vi "WriteDAQ_2AO.vi"(0 "data":dbl format="%0.2f", 1 "array":cluster{dbl, string, "Output Channels":tag}[](array[cluster]), 2 "Channel":i32=1) -> ()   [LabVIEW 2013]
uses:
  <vilib>/DAQmx/write.llb/DAQmx Write (Analog DBL 1Chan 1Samp).vi
  <vilib>/DAQmx/create/channels.llb/DAQmx Create Channel (AO-Voltage-Basic).vi
  <vilib>/DAQmx/miscellaneous.llb/DAQmx Fill In Error Info.vi
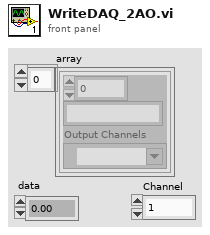
[diagram p1: front panel]
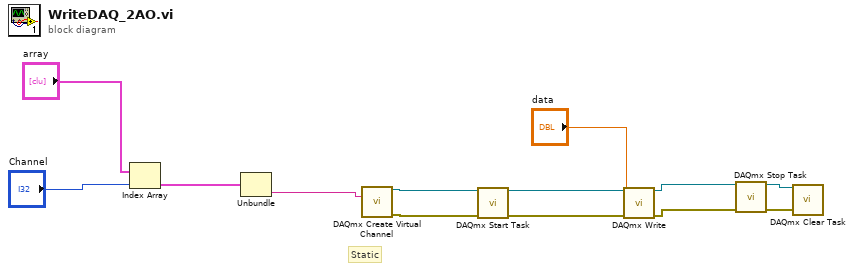
[diagram p0: block diagram]
diagram:
  # "Static"
  n1 = Index Array(array="array", index="Channel") -> (element=w5:cluster{dbl, string, "Output Channels":tag})
  n2 = Unbundle(w5) -> ("Output Channels"=w2:tag)  [unwired: 2 out]
  n3 = call-poly <vilib>:"DAQmx Create Virtual Channel.vi"("physical channels"=w2) -> ("task out"=w6:refnum<k21>, "error out"=w7:errorcluster)  [unwired: 13 in]
  n4 = call <vilib>:"DAQmx Start Task.vi"("task/channels in"=w6, "error in"=w7) -> ("task out"=w8:refnum<k21>, "error out"=w9:errorcluster)  [unwired: 12 in]
  n5 = call-poly <vilib>:"DAQmx Write.vi"("task/channels in"=w8, "data"="data", "error in"=w9) -> ("task out"=w10:refnum<k21>, "error out"=w11:errorcluster)  [unwired: 10 in, 1 out]
  n6 = call <vilib>:"DAQmx Stop Task.vi"("task/channels in"=w10, "error in"=w11) -> ("task out"=w13:refnum<k21>, "error out"=w12:errorcluster)  [unwired: 12 in]
  n7 = call <vilib>:"DAQmx Clear Task.vi"("task in"=w13, "error in"=w12) -> ()  [unwired: 13 in, 1 out]
